vi "Attenuator Determine Limit.vi"(10 "Attenuation Value (0 dB)":dbl min=0.0 max=63.75 step=0.25 format="%.2f") -> (2 "Maximum Error (dB)":dbl)   [LabVIEW 2011]
uses:
  Summitek EXT/OpenG EXT/array/array.llb/Filter 1D Array with Scalar (Boolean)__ogtk.vi
  Summitek EXT/OpenG EXT/array/array.llb/Index 1D Array Elements (DBL)__ogtk.vi
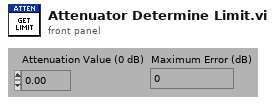
[diagram p1: front panel]
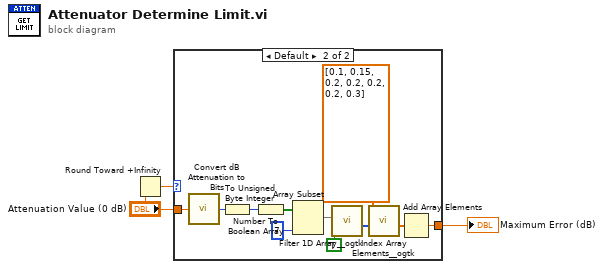
[diagram p0: block diagram]
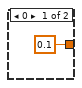
[diagram p2: hidden frame]
diagram:
  n1 = Round Toward +Infinity(x="Attenuation Value (0 dB)") -> (ceil(x): smallest int >= x=w1:dbl)
  n2 = case shown="Default" w1 {
    tunnel: [0.1 w6] -> w3
    tunnel: "Attenuation Value (0 dB)" -> [_ w5]
    frame 0 {
    }
    frame Default {
      n3 = call "Convert dB Attenuation to Bits.vi"("Attenuation Value (0 dB)"=w5) -> ("Binary VA Value"=w13:u32)  [unwired: 4 out]
      n4 = To Unsigned Byte Integer(number=w13) -> (unsigned 8bit integer=w15:u8)
      n5 = Number To Boolean Array(number=w15) -> (Boolean array=w14:bool[])
      n6 = Array Subset(array=w14, length=7) -> (w11:bool[])  [unwired: 1 in]
      n7 = call-poly "Filter 1D Array__ogtk.vi"("items to filter"=TRUE, "array"=w11) -> ("filtered item indices"=w9:i32[])  [unwired: 4 in, 1 out]
      n8 = call-poly "Index Array Elements__ogtk.vi"("indices"=w9, "array"=dbl[] [0.1, 0.15, 0.2, 0.2, 0.2, 0.2, 0.3]) -> ("elements"=w7:dbl[])  [unwired: 9 in]
      n9 = Add Array Elements(numeric array=w7) -> (sum=w6:dbl)
    }
  }
  "Maximum Error (dB)" <- w3
